vi "homework - formula xy graph.vi"() -> ()   [LabVIEW 2024]
doc: "#vi_description \nPlots a polynomial equation to an XY graph, demonstrating the use of a formula node.\nThetic Engineering Ltd."
uses:
  <vilib>/Analysis/1siggen.llb/Ramp Pattern by Samples.vi
  <vilib>/Analysis/NI_AALBase.lvlib
panel:
  out "XY Graph":cluster{"Ramp Pattern":dbl[], dbl[]}(graph)
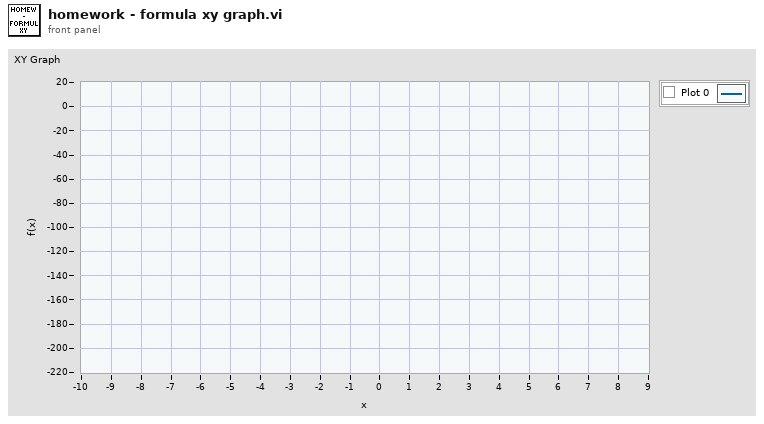
[diagram p1: front panel]
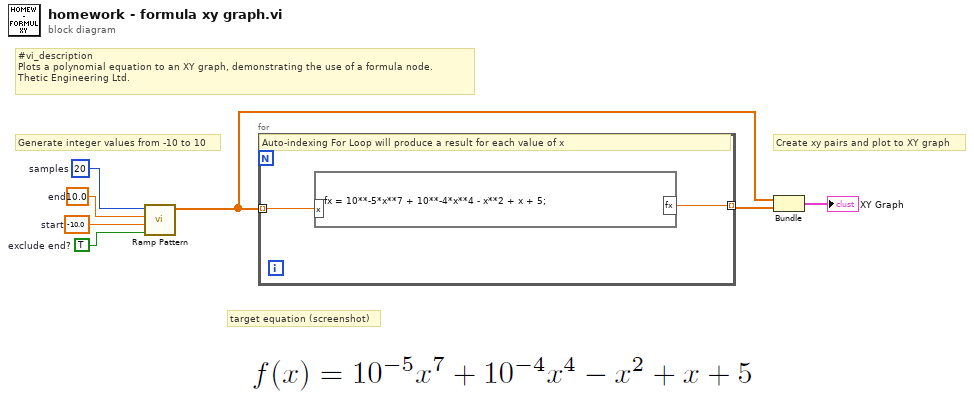
[diagram p0: block diagram]
diagram:
  w1 = TRUE  # exclude end?
  w5 = 20  # samples
  w6 = 10.0  # end
  w7 = -10.0  # start
  # "#vi_description \nPlots a polynomial equation to an XY graph, demonstrating the use of a formula node.\nThetic Engineering Ltd."
  # "Create xy pairs and plot to XY graph"
  # "Generate integer values from -10 to 10"
  # "target equation (screenshot)"
  n1 = call-poly <vilib>:"Ramp Pattern.vi"("exclude end?"=w1, "start"=w7, "end"=w6, "samples"=w5) -> ("Ramp Pattern"=w3:dbl[])  [unwired: 6 in, 1 out]
  n2 = for {
    tunnel: w3 -> [w9] mode=indexing
    tunnel: [w8] -> w4 mode=indexing
    # "Auto-indexing For Loop will produce a result for each value of x"
    n3 = formula code="fx = 10**-5*x**7 + 10**-4*x**4 - x**2 + x + 5;"("x"=w9) -> ("fx"=w8:dbl)
  }
  n4 = Bundle("Ramp Pattern"=w3, w4) -> (→"XY Graph":cluster{"Ramp Pattern":dbl[], dbl[]})  [unwired: 1 in]
